vi "MV3D RGBD Open Device By Serial Number.vi"(10 "chSerialNumber":string, 11 "handle":u32) -> (2 "function return":i32, 3 "handle out":u32)   [LabVIEW 2015, in "Mv3dRgbd.lvlib"]
doc: "MV3D_RGBD_API MV3D_RGBD_STATUS MV3D_RGBD_OpenDeviceBySerialNumber(HANDLE *handle, const char* chSerialNumber);"
uses:
  <userlib>/Mv3dRgbd/Mv3dRgbd.lvlib
  <userlib>/Mv3dRgbd/Mv3dRgbd.dll
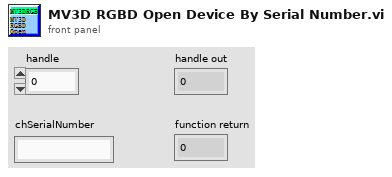
[diagram p1: front panel]
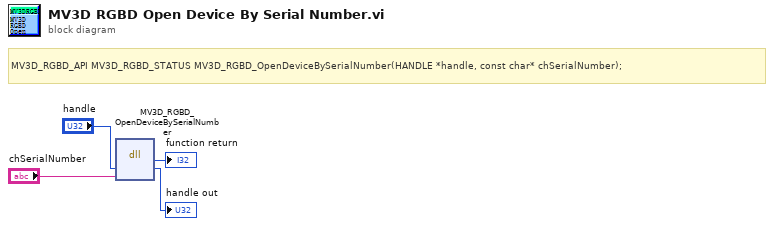
[diagram p0: block diagram]
diagram:
  # "MV3D_RGBD_API MV3D_RGBD_STATUS MV3D_RGBD_OpenDeviceBySerialNumber(HANDLE *handle, const char* chSerialNumber);"
  n1 = dll-call lib="C:/Program Files (x86)/National Instruments/LabVIEW 2015/user.lib/Mv3dRgbd/Mv3dRgbd.*" fn="MV3D_RGBD_OpenDeviceBySerialNumber"("handle"="handle", "chSerialNumber"="chSerialNumber") -> (→"function return":i32, "handle"=→"handle out":u32)  [unwired: 4 in, 2 out]
